vi "staticUpdateHWError.vi"(8 "error in (no error)":errorcluster, 11 "AtomChipHWC in":refnum<class "AtomChipHWC.lvclass">) -> (0 "error out":errorcluster, 3 "AtomChipHWC out":refnum<class "AtomChipHWC.lvclass">)   [LabVIEW 2011, in "Hardware.lvlib" / "HWControllers.lvlib" / "AtomChipHWC.lvclass"]
uses:
  AtomChipHWC.lvclass
  AtomChipHWC.lvclass/AtomChipHWC.ctl
  Channels/Digital/DigitalOutput.lvclass
  Channels/VoltOutput/AnalogOutput.lvclass
  Channels/DDSOutput/Generic/DDSOutput.lvclass
  Network Controllers/CameraNetworkController/CameraNetworkController.lvclass
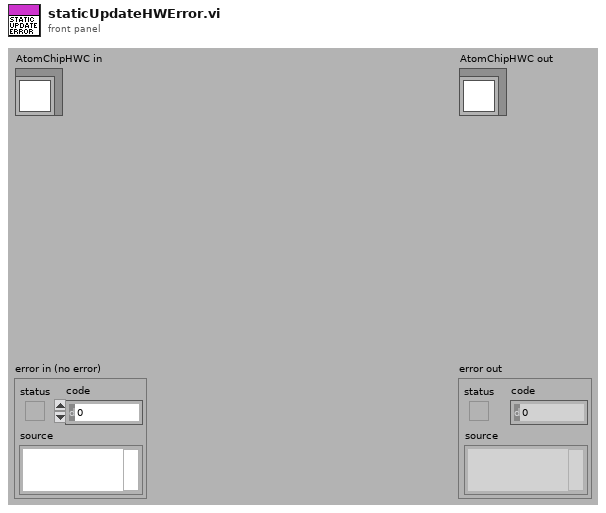
[diagram p1: front panel]
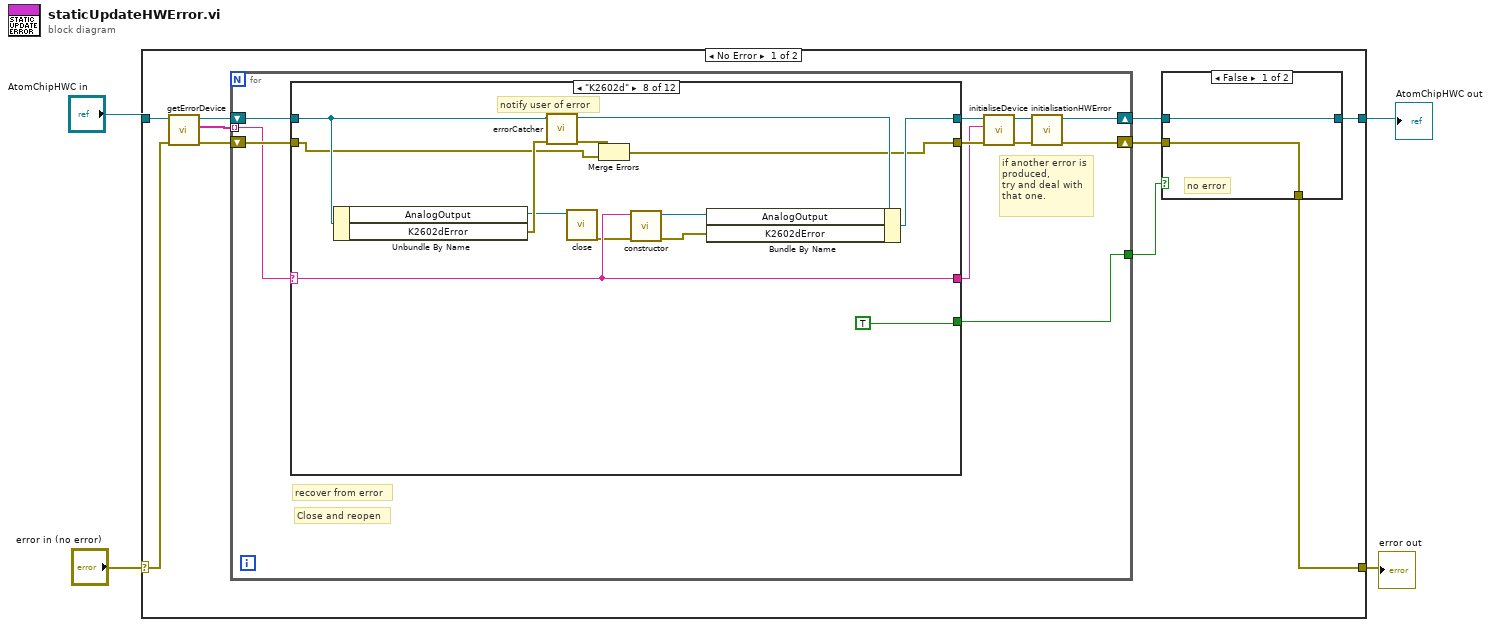
[diagram p0: block diagram]
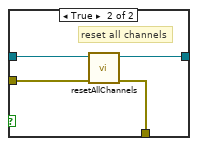
[diagram p2: hidden frame]
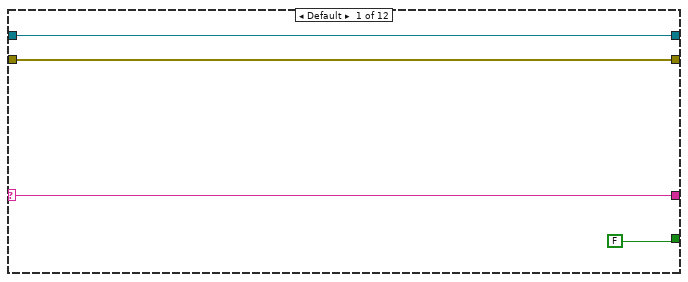
[diagram p3: hidden frame]
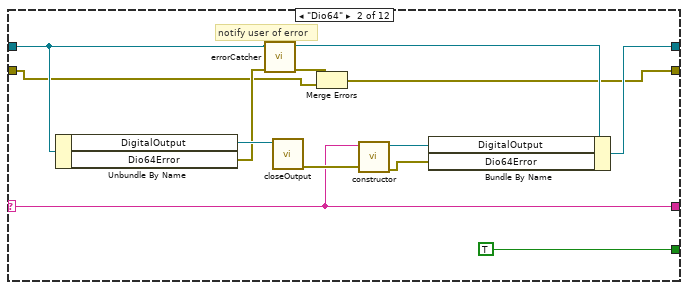
[diagram p4: hidden frame]
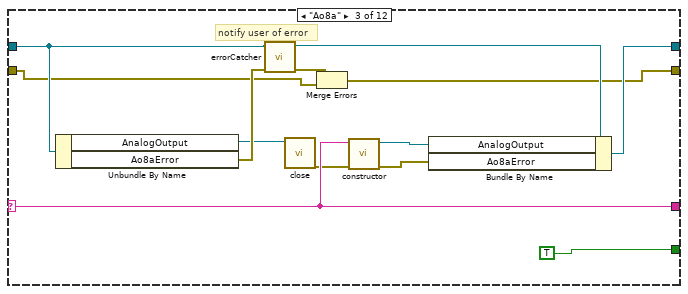
[diagram p5: hidden frame]
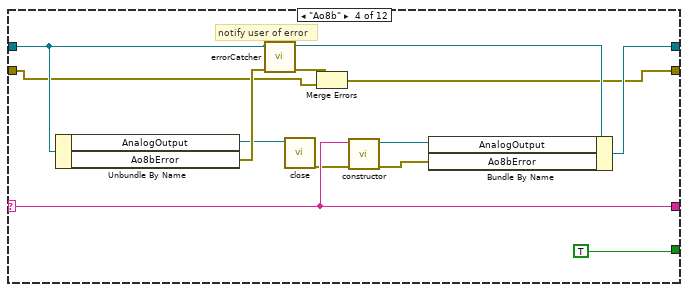
[diagram p6: hidden frame]
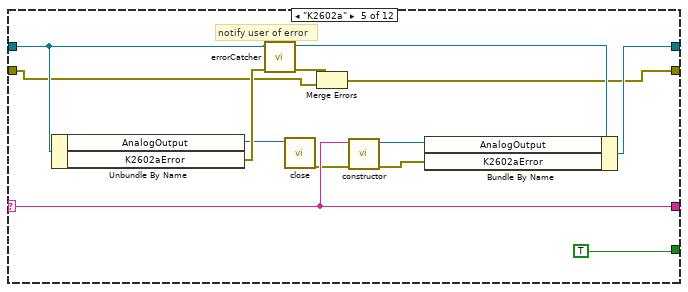
[diagram p7: hidden frame]
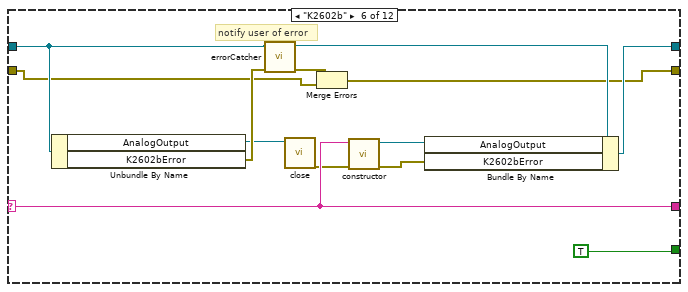
[diagram p8: hidden frame]
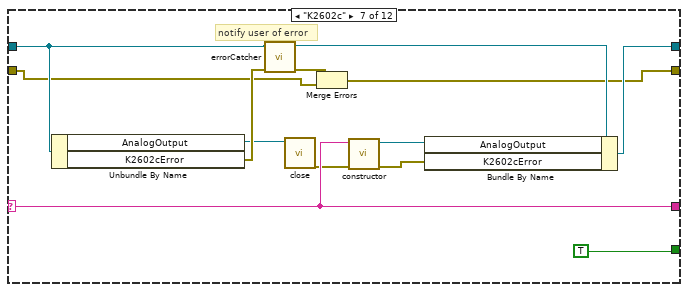
[diagram p9: hidden frame]
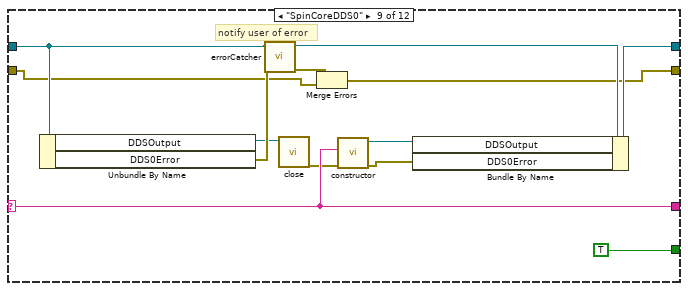
[diagram p10: hidden frame]
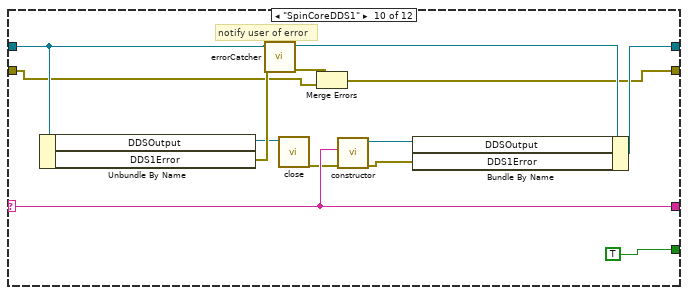
[diagram p11: hidden frame]
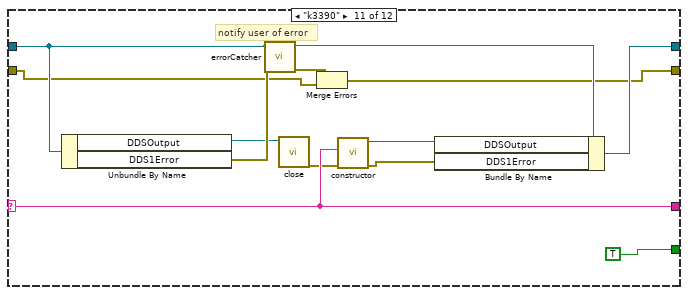
[diagram p12: hidden frame]
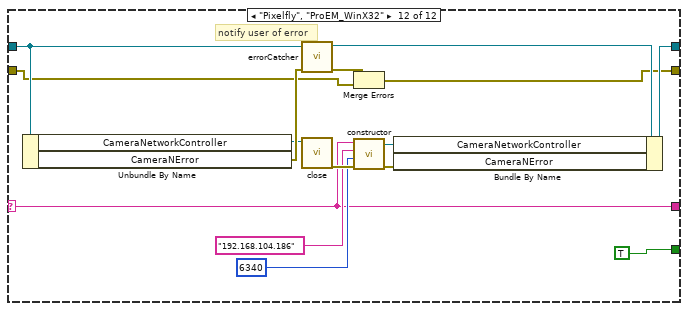
[diagram p13: hidden frame]
diagram:
  n1 = case shown="No Error" "error in (no error)" {
    selector: "error in (no error)" -> [w13 w181]
    tunnel: "AtomChipHWC in" -> [w14 w182]
    tunnel: [w7 w182] -> w2
    tunnel: [w6 w181] -> w1
    frame No Error {
      n2 = call "getErrorDevice.vi"("error in (no error)"=w13, "AtomChipHWC in"=w14) -> ("error out"=w10:errorcluster, "Devices"=w11:string[], "AtomChipHWC out"=w12:refnum<class "AtomChipHWC.lvclass">)  [unwired: 7 in]
      n3 = for {
        tunnel: w11 -> [w29] mode=indexing
        shift-right: [w23] -> w9
        shift-left: w12 -> [w31]
        shift-right: [w22] -> w8
        shift-left: w10 -> [w30]
        tunnel: [w21] -> w5
        # "Close and reopen"
        # "if another error is\nproduced,\ntry and deal with\nthat one."
        # "recover from error"
        n4 = case shown="\"K2602d\"" w29 {
          selector: w29 -> [w33 w37 w53 w66 w79 w92 w105 w118 w129 w142 w155 w167]
          tunnel: w31 -> [w35 w44 w61 w74 w87 w100 w113 w126 w139 w152 w165 w180]
          tunnel: [w35 w39 w56 w69 w82 w95 w108 w121 w134 w147 w160 w175] -> w26
          tunnel: [w34 w38 w55 w68 w81 w94 w107 w120 w133 w146 w159 w174] -> w25
          tunnel: w30 -> [w34 w40 w57 w70 w83 w96 w109 w122 w135 w148 w161 w176]
          tunnel: [w33 w37 w53 w66 w79 w92 w105 w118 w129 w142 w155 w167] -> w24
          tunnel: [FALSE TRUE TRUE TRUE TRUE TRUE TRUE TRUE TRUE TRUE TRUE TRUE] -> w21
          frame Default {
          }
          frame "Dio64" {
            # "notify user of error"
            n5 = Unbundle By Name(w44) -> ("DigitalOutput"=w48:refnum<class "DigitalOutput.lvclass">, "Dio64Error"=w42:errorcluster)
            n6 = call-dynamic "errorCatcher.vi"("error in (no error)"=w42, "HWController in"=w44) -> ("error out"=w41:errorcluster, "HWController out"=w43:refnum<class "AtomChipHWC.lvclass">)  [unwired: 8 in]
            n7 = call-dynamic "closeOutput.vi"("DigitalOutput in"=w48) -> ("error out"=w47:errorcluster)  [unwired: 10 in]
            n8 = Merge Errors(w41, w40) -> (w38:errorcluster)
            n9 = call "constructor.vi"("error in (no error)"=w47, "deviceName"=w37) -> ("error out"=w45:errorcluster, "DigitalOutput out"=w46:refnum<class "DigitalOutput.lvclass">)  [unwired: 8 in]
            n10 = Bundle By Name(cluster=w43, "DigitalOutput"=w46, "Dio64Error"=w45) -> (w39:refnum<class "AtomChipHWC.lvclass">)
          }
          frame "Ao8a" {
            # "notify user of error"
            n11 = Unbundle By Name(w61) -> ("AnalogOutput"=w54:refnum<class "AnalogOutput.lvclass">, "Ao8aError"=w59:errorcluster)
            n12 = call-dynamic "errorCatcher.vi"("error in (no error)"=w59, "HWController in"=w61) -> ("error out"=w58:errorcluster, "HWController out"=w60:refnum<class "AtomChipHWC.lvclass">)  [unwired: 8 in]
            n13 = call-dynamic "close.vi"("AnalogOutput in"=w54) -> ("error out"=w52:errorcluster)  [unwired: 10 in]
            n14 = Merge Errors(w58, w57) -> (w55:errorcluster)
            n15 = call "constructor.vi"("error in (no error)"=w52, "deviceName"=w53) -> ("error out"=w50:errorcluster, "AnalogOutput out"=w51:refnum<class "AnalogOutput.lvclass">)  [unwired: 8 in]
            n16 = Bundle By Name(cluster=w60, "AnalogOutput"=w51, "Ao8aError"=w50) -> (w56:refnum<class "AtomChipHWC.lvclass">)
          }
          frame "Ao8b" {
            # "notify user of error"
            n17 = Unbundle By Name(w74) -> ("AnalogOutput"=w67:refnum<class "AnalogOutput.lvclass">, "Ao8bError"=w72:errorcluster)
            n18 = call-dynamic "errorCatcher.vi"("error in (no error)"=w72, "HWController in"=w74) -> ("error out"=w71:errorcluster, "HWController out"=w73:refnum<class "AtomChipHWC.lvclass">)  [unwired: 8 in]
            n19 = call-dynamic "close.vi"("AnalogOutput in"=w67) -> ("error out"=w65:errorcluster)  [unwired: 10 in]
            n20 = Merge Errors(w71, w70) -> (w68:errorcluster)
            n21 = call "constructor.vi"("error in (no error)"=w65, "deviceName"=w66) -> ("error out"=w63:errorcluster, "AnalogOutput out"=w64:refnum<class "AnalogOutput.lvclass">)  [unwired: 8 in]
            n22 = Bundle By Name(cluster=w73, "AnalogOutput"=w64, "Ao8bError"=w63) -> (w69:refnum<class "AtomChipHWC.lvclass">)
          }
          frame "K2602a" {
            # "notify user of error"
            n23 = Unbundle By Name(w87) -> ("AnalogOutput"=w80:refnum<class "AnalogOutput.lvclass">, "K2602aError"=w85:errorcluster)
            n24 = call-dynamic "errorCatcher.vi"("error in (no error)"=w85, "HWController in"=w87) -> ("error out"=w84:errorcluster, "HWController out"=w86:refnum<class "AtomChipHWC.lvclass">)  [unwired: 8 in]
            n25 = call-dynamic "close.vi"("AnalogOutput in"=w80) -> ("error out"=w78:errorcluster)  [unwired: 10 in]
            n26 = Merge Errors(w84, w83) -> (w81:errorcluster)
            n27 = call "constructor.vi"("error in (no error)"=w78, "deviceName"=w79) -> ("error out"=w76:errorcluster, "AnalogOutput out"=w77:refnum<class "AnalogOutput.lvclass">)  [unwired: 8 in]
            n28 = Bundle By Name(cluster=w86, "AnalogOutput"=w77, "K2602aError"=w76) -> (w82:refnum<class "AtomChipHWC.lvclass">)
          }
          frame "K2602b" {
            # "notify user of error"
            n29 = Unbundle By Name(w100) -> ("AnalogOutput"=w93:refnum<class "AnalogOutput.lvclass">, "K2602bError"=w98:errorcluster)
            n30 = call-dynamic "errorCatcher.vi"("error in (no error)"=w98, "HWController in"=w100) -> ("error out"=w97:errorcluster, "HWController out"=w99:refnum<class "AtomChipHWC.lvclass">)  [unwired: 8 in]
            n31 = call-dynamic "close.vi"("AnalogOutput in"=w93) -> ("error out"=w91:errorcluster)  [unwired: 10 in]
            n32 = Merge Errors(w97, w96) -> (w94:errorcluster)
            n33 = call "constructor.vi"("error in (no error)"=w91, "deviceName"=w92) -> ("error out"=w89:errorcluster, "AnalogOutput out"=w90:refnum<class "AnalogOutput.lvclass">)  [unwired: 8 in]
            n34 = Bundle By Name(cluster=w99, "AnalogOutput"=w90, "K2602bError"=w89) -> (w95:refnum<class "AtomChipHWC.lvclass">)
          }
          frame "K2602c" {
            # "notify user of error"
            n35 = Unbundle By Name(w113) -> ("AnalogOutput"=w106:refnum<class "AnalogOutput.lvclass">, "K2602cError"=w111:errorcluster)
            n36 = call-dynamic "errorCatcher.vi"("error in (no error)"=w111, "HWController in"=w113) -> ("error out"=w110:errorcluster, "HWController out"=w112:refnum<class "AtomChipHWC.lvclass">)  [unwired: 8 in]
            n37 = call-dynamic "close.vi"("AnalogOutput in"=w106) -> ("error out"=w104:errorcluster)  [unwired: 10 in]
            n38 = Merge Errors(w110, w109) -> (w107:errorcluster)
            n39 = call "constructor.vi"("error in (no error)"=w104, "deviceName"=w105) -> ("error out"=w102:errorcluster, "AnalogOutput out"=w103:refnum<class "AnalogOutput.lvclass">)  [unwired: 8 in]
            n40 = Bundle By Name(cluster=w112, "AnalogOutput"=w103, "K2602cError"=w102) -> (w108:refnum<class "AtomChipHWC.lvclass">)
          }
          frame "K2602d" {
            # "notify user of error"
            n41 = Unbundle By Name(w126) -> ("AnalogOutput"=w119:refnum<class "AnalogOutput.lvclass">, "K2602dError"=w124:errorcluster)
            n42 = call-dynamic "errorCatcher.vi"("error in (no error)"=w124, "HWController in"=w126) -> ("error out"=w123:errorcluster, "HWController out"=w125:refnum<class "AtomChipHWC.lvclass">)  [unwired: 8 in]
            n43 = call-dynamic "close.vi"("AnalogOutput in"=w119) -> ("error out"=w117:errorcluster)  [unwired: 10 in]
            n44 = Merge Errors(w123, w122) -> (w120:errorcluster)
            n45 = call "constructor.vi"("error in (no error)"=w117, "deviceName"=w118) -> ("error out"=w115:errorcluster, "AnalogOutput out"=w116:refnum<class "AnalogOutput.lvclass">)  [unwired: 8 in]
            n46 = Bundle By Name(cluster=w125, "AnalogOutput"=w116, "K2602dError"=w115) -> (w121:refnum<class "AtomChipHWC.lvclass">)
          }
          frame "SpinCoreDDS0" {
            # "notify user of error"
            n47 = Unbundle By Name(w139) -> ("DDSOutput"=w132:refnum<class "DDSOutput.lvclass">, "DDS0Error"=w137:errorcluster)
            n48 = call-dynamic "errorCatcher.vi"("error in (no error)"=w137, "HWController in"=w139) -> ("error out"=w136:errorcluster, "HWController out"=w138:refnum<class "AtomChipHWC.lvclass">)  [unwired: 8 in]
            n49 = call-dynamic "close.vi"("DDSOutput in"=w132) -> ("error out"=w128:errorcluster)  [unwired: 10 in]
            n50 = Merge Errors(w136, w135) -> (w133:errorcluster)
            n51 = call "constructor.vi"("error in (no error)"=w128, "device"=w129) -> ("error out"=w130:errorcluster, "DDSOutput out"=w131:refnum<class "DDSOutput.lvclass">)  [unwired: 8 in]
            n52 = Bundle By Name(cluster=w138, "DDSOutput"=w131, "DDS0Error"=w130) -> (w134:refnum<class "AtomChipHWC.lvclass">)
          }
          frame "SpinCoreDDS1" {
            # "notify user of error"
            n53 = Unbundle By Name(w152) -> ("DDSOutput"=w145:refnum<class "DDSOutput.lvclass">, "DDS1Error"=w150:errorcluster)
            n54 = call-dynamic "errorCatcher.vi"("error in (no error)"=w150, "HWController in"=w152) -> ("error out"=w149:errorcluster, "HWController out"=w151:refnum<class "AtomChipHWC.lvclass">)  [unwired: 8 in]
            n55 = call-dynamic "close.vi"("DDSOutput in"=w145) -> ("error out"=w141:errorcluster)  [unwired: 10 in]
            n56 = Merge Errors(w149, w148) -> (w146:errorcluster)
            n57 = call "constructor.vi"("error in (no error)"=w141, "device"=w142) -> ("error out"=w143:errorcluster, "DDSOutput out"=w144:refnum<class "DDSOutput.lvclass">)  [unwired: 8 in]
            n58 = Bundle By Name(cluster=w151, "DDSOutput"=w144, "DDS1Error"=w143) -> (w147:refnum<class "AtomChipHWC.lvclass">)
          }
          frame "k3390" {
            # "notify user of error"
            n59 = Unbundle By Name(w165) -> ("DDSOutput"=w158:refnum<class "DDSOutput.lvclass">, "DDS1Error"=w163:errorcluster)
            n60 = call-dynamic "errorCatcher.vi"("error in (no error)"=w163, "HWController in"=w165) -> ("error out"=w162:errorcluster, "HWController out"=w164:refnum<class "AtomChipHWC.lvclass">)  [unwired: 8 in]
            n61 = call-dynamic "close.vi"("DDSOutput in"=w158) -> ("error out"=w154:errorcluster)  [unwired: 10 in]
            n62 = Merge Errors(w162, w161) -> (w159:errorcluster)
            n63 = call "constructor.vi"("error in (no error)"=w154, "device"=w155) -> ("error out"=w156:errorcluster, "DDSOutput out"=w157:refnum<class "DDSOutput.lvclass">)  [unwired: 8 in]
            n64 = Bundle By Name(cluster=w164, "DDSOutput"=w157, "DDS1Error"=w156) -> (w160:refnum<class "AtomChipHWC.lvclass">)
          }
          frame "Pixelfly", "ProEM_WinX32" {
            # "notify user of error"
            n65 = Unbundle By Name(w180) -> ("CameraNetworkController"=w173:refnum<class "CameraNetworkController.lvclass">, "CameraNError"=w178:errorcluster)
            n66 = call-dynamic "errorCatcher.vi"("error in (no error)"=w178, "HWController in"=w180) -> ("error out"=w177:errorcluster, "HWController out"=w179:refnum<class "AtomChipHWC.lvclass">)  [unwired: 8 in]
            n67 = call "close.vi"("CameraNetworkController in"=w173) -> ("error out"=w170:errorcluster)  [unwired: 9 in, 1 out]
            n68 = Merge Errors(w177, w176) -> (w174:errorcluster)
            n69 = call "constructor.vi"("error in (no error)"=w170, "remote port"=u16 6340, "remote address"="192.168.104.186", "camera"=w167) -> ("error out"=w171:errorcluster, "CameraNetworkController out"=w172:refnum<class "CameraNetworkController.lvclass">)  [unwired: 6 in]
            n70 = Bundle By Name(cluster=w179, "CameraNetworkController"=w172, "CameraNError"=w171) -> (w175:refnum<class "AtomChipHWC.lvclass">)
          }
        }
        n71 = call "initialiseDevice.vi"("error in (no error)"=w25, "deviceName"=w24, "AtomChipHWC in"=w26) -> ("error out"=w27:errorcluster, "AtomChipHWC out"=w28:refnum<class "AtomChipHWC.lvclass">)  [unwired: 7 in]
        n72 = call-dynamic "initialisationHWError.vi"("error in (no error)"=w27, "AtomChipHWC in"=w28) -> ("error out"=w22:errorcluster, "AtomChipHWC out"=w23:refnum<class "AtomChipHWC.lvclass">)  [unwired: 8 in]
      }
      n73 = case shown="False" w5 {
        tunnel: w9 -> [w16 w20]
        tunnel: w8 -> [w15 w19]
        tunnel: [w16 w18] -> w7
        tunnel: [w15 w17] -> w6
        frame False {
          # "no error"
        }
        frame True {
          # "reset all channels"
          n74 = call-dynamic "resetAllChannels.vi"("error in (no error)"=w19, "AtomChipHWC in"=w20) -> ("error out"=w17:errorcluster, "AtomChipHWC out"=w18:refnum<class "AtomChipHWC.lvclass">)  [unwired: 8 in]
        }
      }
    }
    frame Error {
    }
  }
  "error out" <- w1
  "AtomChipHWC out" <- w2
